vi "GenerateAttachablePosition_King.vi"(1 "Castling State":bool[][](array[boolean]), 2 "Black/White Turn (T/F)":bool, 3 "pieceIndex":i32, 4 "Board":i32[][](array[numeric])=[[-3, -5, -4, -1, -2, -4, -5, -3], [-6, -6, -6, -6, -6, -6, -6, -6], [0, 0, 0, 0, 0, 0, 0, 0], [0, 0, 0, 0, 0, 0, 0, 0], [0, 0, 0, 0, 0, 0, 0, 0], [0, 0, 0, 0, 0, 0, 0, 0], [6, 6, 6, 6, 6, 6, 6, 6], [3, 5, 4, 1, 2, 4, 5, 3]]) -> (0 "AttachablePosition":bool[][](array[boolean]))   [LabVIEW 2014]
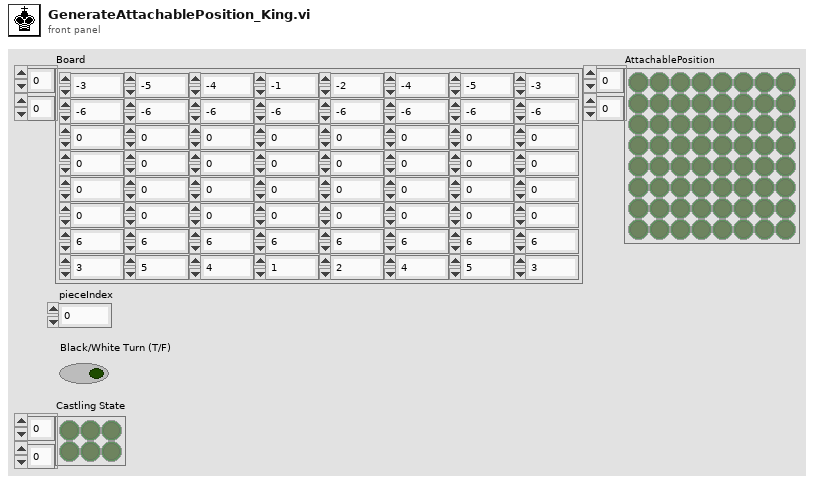
[diagram p1: front panel]
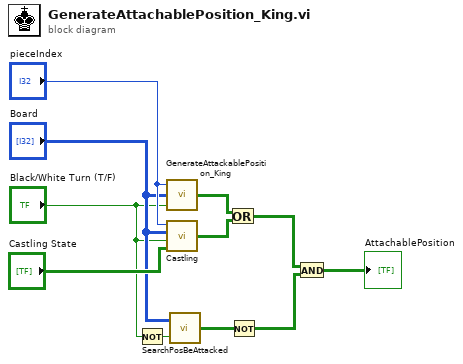
[diagram p0: block diagram]
diagram:
  n1 = Not(x="Black/White Turn (T/F)") -> (.not. x?=w7:bool)
  n2 = call "GenerateAttackablePosition_King.vi"("Black/White Turn (T/F)"="Black/White Turn (T/F)", "Board"="Board", "pieceIndex"="pieceIndex") -> ("AttackablePosition"=w5:bool[][])
  n3 = call "Castling.vi"("Castling State"="Castling State", "Black/White Turn (T/F)"="Black/White Turn (T/F)", "Board"="Board", "pieceIndex"="pieceIndex") -> ("Castling position"=w6:bool[][])
  n4 = call "SearchPosBeAttacked.vi"("Black/White (T/F)"=w7, "Board"="Board") -> ("AttackablePosition"=w4:bool[][])
  n5 = Or(x=w5, y=w6) -> (x .or. y?=w2:bool[][])
  n6 = Not(x=w4) -> (.not. x?=w3:bool[][])
  n7 = And(x=w2, y=w3) -> (x .and. y?=→"AttachablePosition":bool[][])
